vi "RichToFlatni_xnet_can_bm_api_GetStreamingFilterRequest.vi"(5 "OutputClusterType":T1, 11 "InputCluster":T3) -> (3 "OutputCluster":T1)   [LabVIEW 2025, in "xnet_can_bus_monitor_api_client.lvlib"]
uses:
  xnet_can_bus_monitor_api_client.lvlib
  ni_xnet_can_bm_api_GetStreamingFilterRequest.ctl
  ni_xnet_can_bm_api_Session.ctl
  ni_xnet_can_bm_api_GetStreamingFilterRequest_Flat.ctl
  ni_xnet_can_bm_api_Session_Flat.ctl
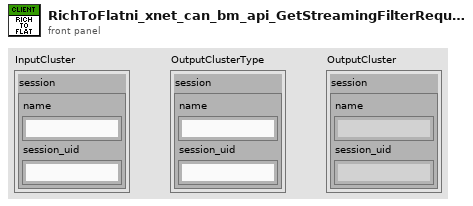
[diagram p1: front panel]
types:
  T1 = typedef "xnet_can_bus_monitor_api_client.lvlib/ni_xnet_can_bm_api_GetStreamingFilterRequest_Flat.ctl" = cluster{"session":T2}
  T2 = typedef "xnet_can_bus_monitor_api_client.lvlib/ni_xnet_can_bm_api_Session_Flat.ctl" = cluster{"name":string, "session_uid":string}
  T3 = typedef "xnet_can_bus_monitor_api_client.lvlib/ni_xnet_can_bm_api_GetStreamingFilterRequest.ctl" = cluster{"session":T4}
  T4 = typedef "xnet_can_bus_monitor_api_client.lvlib/ni_xnet_can_bm_api_Session.ctl" = cluster{"name":string, "session_uid":string}
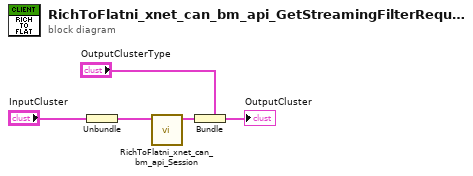
[diagram p0: block diagram]
diagram:
  n1 = Unbundle "Unbundle"("InputCluster") -> ("session"=w2:T4)
  n2 = call "RichToFlatni_xnet_can_bm_api_Session.vi"("InputCluster"=w2) -> ("OutputCluster"=w1:T2)  [unwired: 10 in]
  n3 = Bundle "Bundle"(cluster="OutputClusterType", "session"=w1) -> (→"OutputCluster":T1)
